vi "ADS1293_ECG.vi"() -> ()   [LabVIEW 2019]
uses:
  <vilib>/Analysis/3filter.llb/Filter Passband Type.ctl
  <vilib>/myRIO/Instrument Drivers/Onboard IO/DIO/typedefs/DIO Reference.ctl
  <vilib>/myRIO/Common/Instrument Driver Framework/Utilities/typedefs/myRIO Generic Hardware Reference.ctl
  <vilib>/myRIO/Common/Instrument Driver Framework/Utilities/typedefs/Hardware Version Enum.ctl
  <vilib>/myRIO/Common/Instrument Driver Framework/Utilities/typedefs/myRIO v1.0 Reference.ctl
  <vilib>/myRIO/Common/Instrument Driver Framework/Utilities/typedefs/Generic FPGA Reference.ctl
  <vilib>/myRIO/Common/Instrument Driver Framework/myRIO v1.0/DIO/typedefs/DIO Channels List.ctl
  <vilib>/myRIO/Common/Instrument Driver Framework/myRIO v1.0/DIO/typedefs/DIO Channels Enum.ctl
  <vilib>/userDefined/High Color/nirio_resource_hc.ctl
  <vilib>/myRIO/Instrument Drivers/Onboard IO/SPI/typedefs/SPI User Configuration.ctl
  <vilib>/myRIO/Common/Instrument Driver Framework/myRIO v1.0/SPI/typedefs/SPI Clock Phase.ctl
  <vilib>/myRIO/Common/Instrument Driver Framework/myRIO v1.0/SPI/typedefs/SPI Clock Polarity.ctl
  <vilib>/myRIO/Common/Instrument Driver Framework/myRIO v1.0/SPI/typedefs/SPI Data Direction.ctl
  <vilib>/myRIO/Common/Instrument Driver Framework/myRIO v1.0/SPI/typedefs/SPI Frame Length.ctl
  <vilib>/myRIO/Instrument Drivers/Onboard IO/SPI/typedefs/SPI Reference.ctl
  <vilib>/myRIO/Common/Instrument Driver Framework/myRIO v1.0/SPI/typedefs/SPI Channels Enum.ctl
  <vilib>/myRIO/Instrument Drivers/Onboard IO/SPI/typedefs/SPI Configuration.ctl
  <vilib>/myRIO/Common/Instrument Driver Framework/Utilities/vis/Is FPGA Ref Available.vi
  <vilib>/myRIO/Common/Instrument Driver Framework/myRIO v1.0/DIO/vis/myRIO v1.1 Open DIO.vi
  <vilib>/myRIO/Instrument Drivers/Onboard IO/DIO/vis/Write.vi
  <vilib>/myRIO/Common/Instrument Driver Framework/myRIO v1.0/SPI/vis/myRIO v1.1 Open SPI.vi
  <vilib>/myRIO/Instrument Drivers/Onboard IO/SPI/vis/Configure.vi
  <vilib>/myRIO/Instrument Drivers/Onboard IO/SPI/vis/Write.vi
  <vilib>/myRIO/Instrument Drivers/Onboard IO/SPI/vis/Read.vi
  <vilib>/myRIO/Common/Instrument Driver Framework/Utilities/vis/Validate Channels.vi
  <vilib>/myRIO/Common/Instrument Driver Framework/myRIO v1.0/DIO/vis/myRIO v1.0 Reserve DIO.vi
  <vilib>/myRIO/Common/Instrument Driver Framework/myRIO v1.0/SPI/vis/myRIO v1.0 Reserve SPI.vi
  <vilib>/myRIO/Instrument Drivers/Onboard IO/SPI/vis/Write Read.vi
  <vilib>/myRIO/Common/Instrument Driver Framework/myRIO v1.0/Resource Manager/vis/myRIO v1.0 Reserve Channel List.vi
  <vilib>/myRIO/Common/Instrument Driver Framework/myRIO v1.0/DIO/vis/myRIO v1.0 Build MUX Configuration DIO.vi
  <vilib>/myRIO/Common/Instrument Driver Framework/myRIO v1.0/SPI/vis/myRIO v1.0 Build MUX Configuration SPI.vi
  <vilib>/myRIO/Common/Instrument Driver Framework/myRIO v1.0/Resource Manager/vis/myRIO v1.0 Reserve Channel.vi
  <vilib>/myRIO/Common/Instrument Driver Framework/myRIO v1.0/Resource Manager/vis/myRIO v1.0 Unreserve Channel.vi
  <vilib>/myRIO/Common/Instrument Driver Framework/myRIO v1.0/Resource Manager/vis/myRIO v1.0 Create Configuration List.vi
  <vilib>/myRIO/Common/Instrument Driver Framework/myRIO v1.0/Resource Manager/vis/myRIO v1.0 Build Mutex Name.vi
  <vilib>/Utility/VariantDataType/GetNumericInfo.vi
  <vilib>/Utility/error.llb/Error Cluster From Error Code.vi
  <vilib>/myRIO/Common/Instrument Driver Framework/myRIO v1.0/myRIO v1.1 Open.vi
  <vilib>/myRIO/Common/Instrument Driver Framework/Utilities/vis/IO Manager.vi
  <vilib>/myRIO/Common/Instrument Driver Framework/Utilities/vis/Configuration Manager.vi
  <vilib>/myRIO/Common/Instrument Driver Framework/myRIO v1.0/Resource Manager/vis/myRIO v1.0 Configure IO.vi
  <vilib>/myRIO/Common/Instrument Driver Framework/myRIO v1.0/myRIO v1.0 Close.vi
  <vilib>/myRIO/Common/Instrument Driver Framework/myRIO v1.0/DIO/vis/myRIO v1.0 Write DIO.vi
  <vilib>/myRIO/Common/Instrument Driver Framework/myRIO v1.0/SPI/vis/myRIO v1.0 Configure SPI.vi
  <vilib>/myRIO/Common/Instrument Driver Framework/myRIO v1.0/SPI/vis/myRIO v1.0 Write Read SPI.vi
  <vilib>/myRIO/Express VI/Onboard IO/DO/DO Express VI.xnode
  <vilib>/myRIO/Instrument Drivers/Onboard IO/DIO/vis/myRIO DIO Open.xnode
  <vilib>/myRIO/Express VI/Onboard IO/SPI/SPI Express VI.xnode
  <vilib>/myRIO/Instrument Drivers/Onboard IO/SPI/vis/myRIO SPI Open.xnode
  <vilib>/Analysis/3filter.llb/FIR Windowed Filter (DBL).vi
  <vilib>/myRIO/Instrument Drivers/Onboard IO/SPI/SPI.lvlib
  <vilib>/myRIO/Instrument Drivers/Onboard IO/DIO/DIO.lvlib
  <vilib>/ptbypt/NI_PtbyPt.lvlib
  <vilib>/Analysis/NI_AALBase.lvlib
panel:
  out "OUT 2":waveform(dbl)(graph)
  in  "taps":i32=25 min=1
  in  "sampling freq: fs":dbl=1.0 format="%0.2f"
  in  "filter type":T1
  out "OUT":waveform(dbl)(graph)
  out "Waveform Channel 2":dbl[](graph)
  out "ECG DATA":u16[](array[numeric]) format="%x"
  out "Waveform Channel 1":dbl[](graph)
  out "Channel 2":u32 format="%x"
  out "Channel 1":u32 format="%x"
  in  "N":u32=6
  in  "Read Command":u16[](array[numeric])=[182, 1] format="%x"
  out "Slide":dbl(slide)=inf scale=0.0..1.0
  out "ELAPSED TIME":dbl=0.399439
  in  "SET TIME":dbl=10.0
  in  "CONFIG":u16[](array[numeric])=[0, 1] format="%x"
  in  "CH_CNFG":u16[](array[numeric])=[47, 48] format="%x"
  in  "DRDYB_SRC":u16[](array[numeric])=[39, 8] format="%x"
  in  "R3_RATE_CH2":u16[](array[numeric])=[35, 2] format="%x"
  in  "R3_RATE_CH1":u16[](array[numeric])=[34, 2] format="%x"
  in  "R2_RATE":u16[](array[numeric])=[33, 2] format="%x"
  in  "AFE_SHDN_CN":u16[](array[numeric])=[20, 36] format="%x"
  in  "OSC_CN":u16[](array[numeric])=[18, 4] format="%x"
  in  "RLD_CN":u16[](array[numeric])=[12, 4] format="%x"
  in  "CMDET_EN":u16[](array[numeric])=[10, 7] format="%x"
  in  "FLEX_CH2_CN":u16[](array[numeric])=[2, 25] format="%x"
  in  "FLEX_CH1_CN":u16[](array[numeric])=[1, 17] format="%x"
  # "INITIAL CONFIGURATIONS"
  # "3"
  # "1"
  # "2"
  # "6"
  # "4"
  # "5"
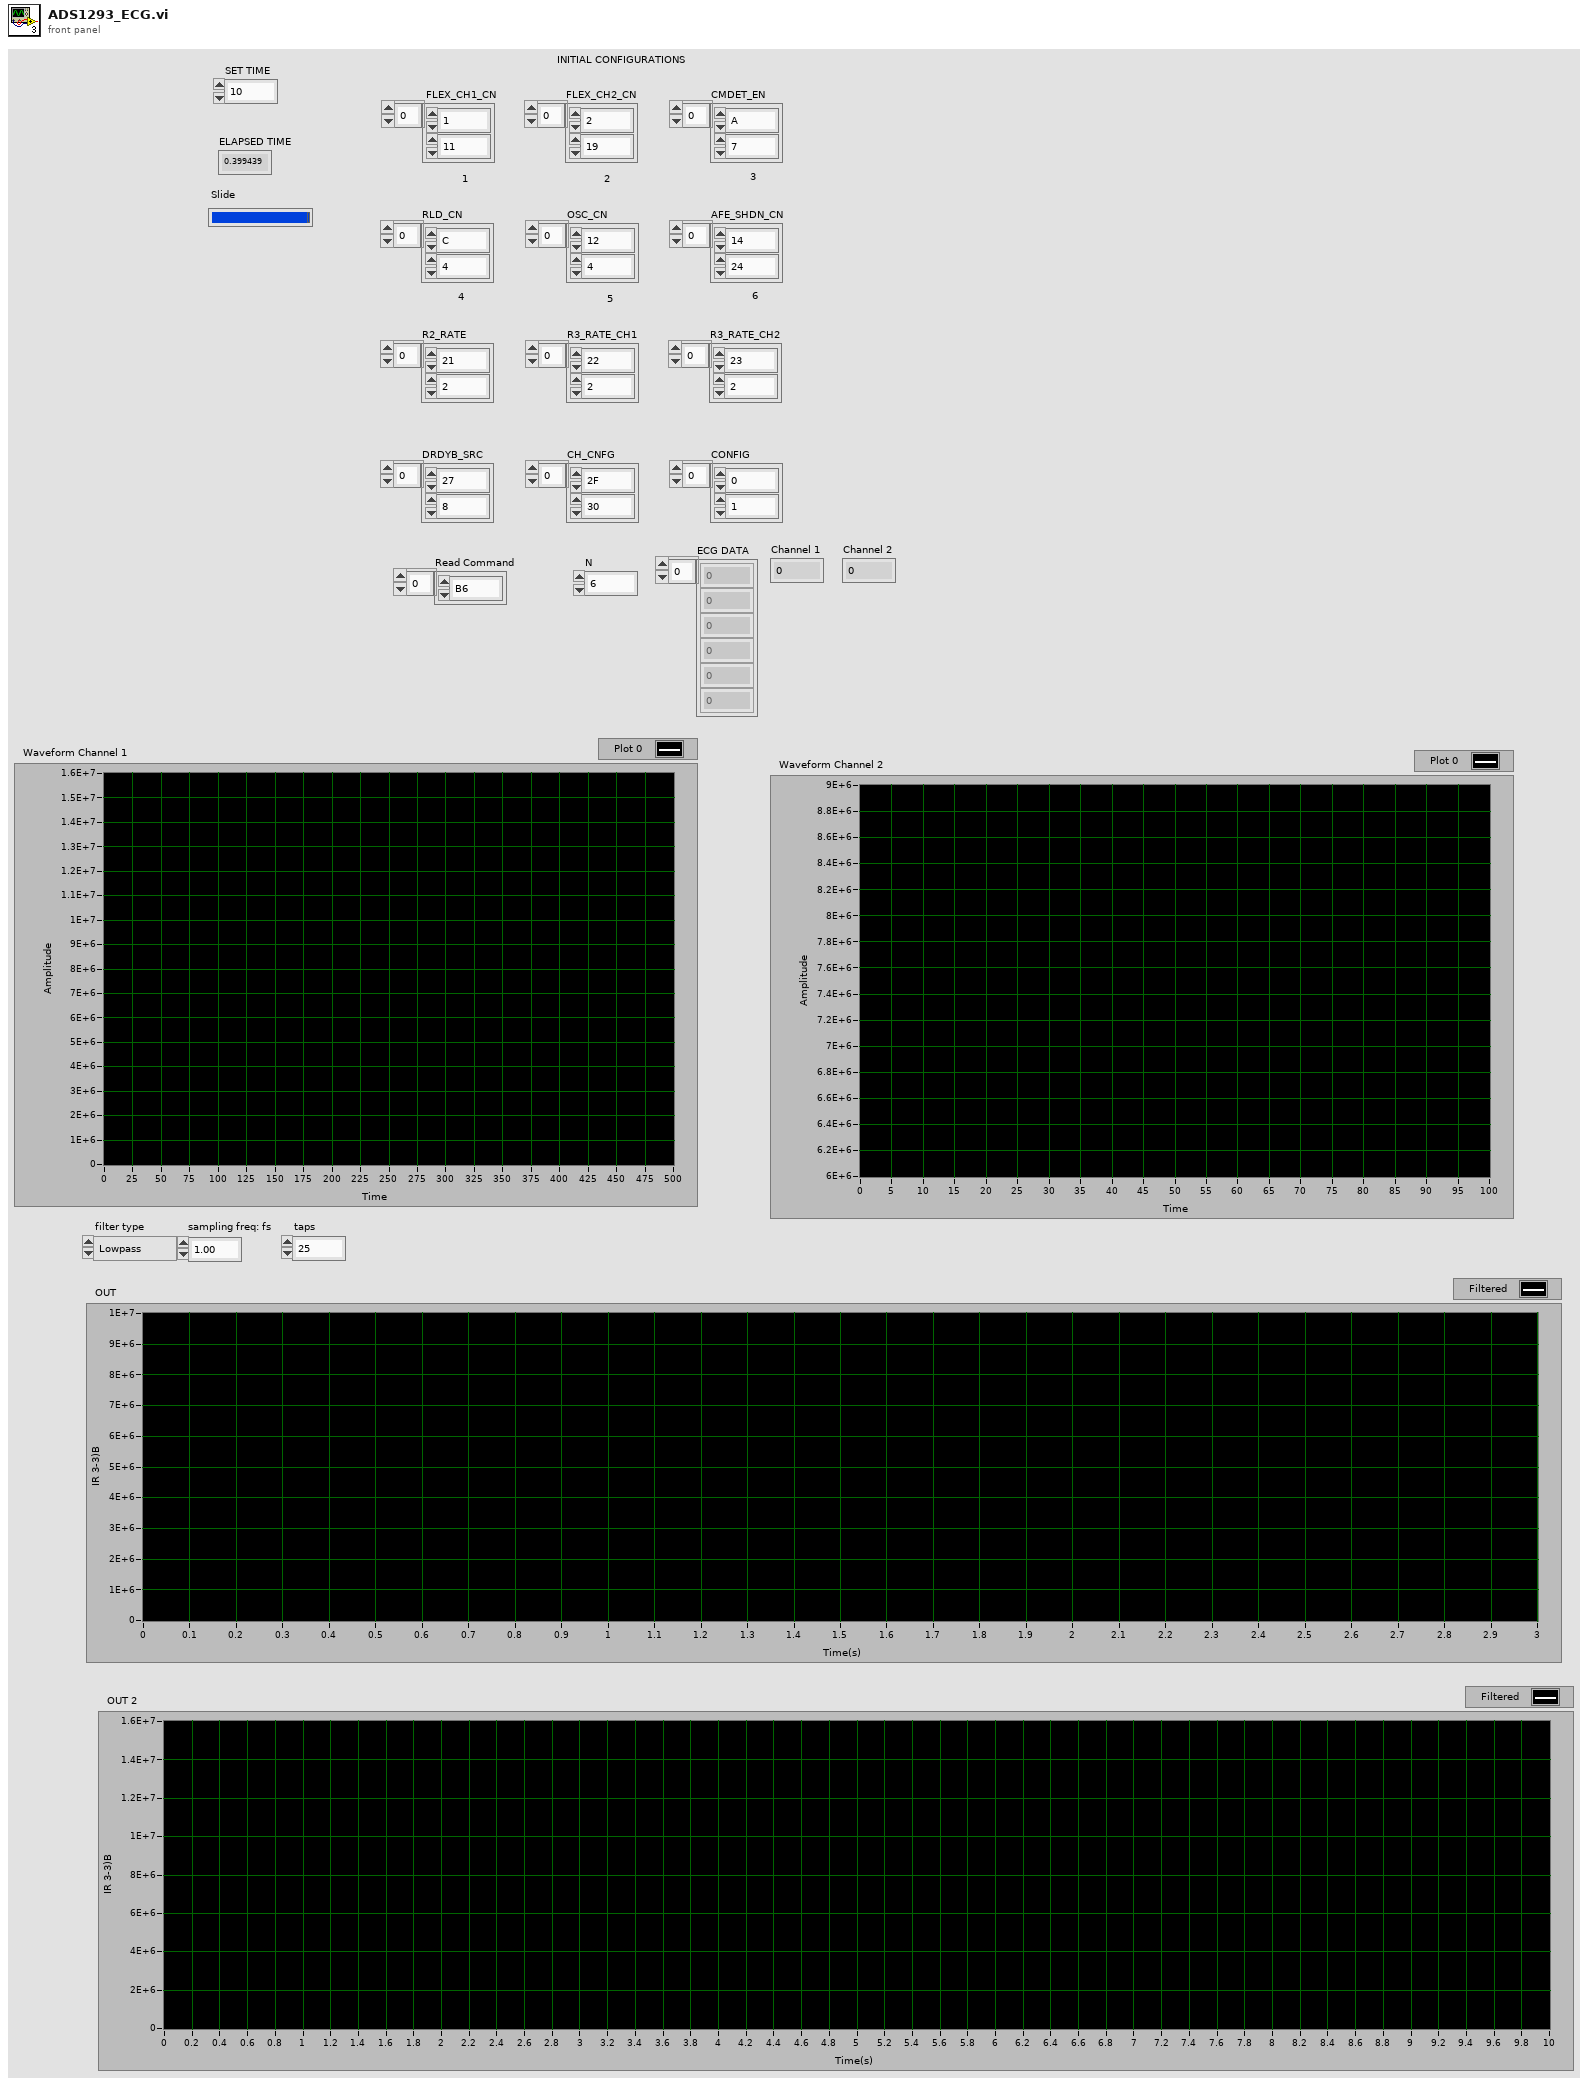
[diagram p1: front panel]
types:
  T1 = typedef "NI_AALBase.lvlib/Filter Passband Type.ctl" = enum32{"Lowpass", "Highpass", "Bandpass", "Bandstop"}
  T2 = typedef "SPI.lvlib/SPI Reference.ctl" = cluster{"myRIO Reference":T3, "SPI Channels Enum":T7, "SPI Configuration":T8}
  T3 = typedef "myRIO Generic Hardware Reference.ctl" = cluster{"myRIO Model":T4, "myRIO Hardware Reference":T5}
  T4 = typedef "Hardware Version Enum.ctl" = enum16{"Unknown", "myRIO-1900", "myRIO-1950", "roboRIO", "NI ELVIS RIO CM", "ELVIS III"}
  T5 = typedef "myRIO v1.0 Reference.ctl" = cluster{"Generic FPGA Reference":T6, "Allow multiple opens":bool}
  T6 = typedef "Generic FPGA Reference.ctl" = refnum<k20>
  T7 = typedef "SPI Channels Enum.ctl" = enum16{"Not Connected", "A/SPI", "B/SPI", "SPI/SPI"}
  T8 = typedef "SPI.lvlib/SPI Configuration.ctl" = cluster{"Frequency [Hz]":dbl, "Clock Phase":T9, "Clock Polarity":T10, "Data Direction":T11, "Frame Length":T12}
  T9 = typedef "SPI Clock Phase.ctl" = enum8{"Leading", "Trailing"}
  T10 = typedef "SPI Clock Polarity.ctl" = enum8{"Low", "High"}
  T11 = typedef "SPI Data Direction.ctl" = enum8{"Most significant bit first", "Least significant bit first"}
  T12 = typedef "SPI Frame Length.ctl" = u8
  T13 = typedef "SPI.lvlib/SPI User Configuration.ctl" = cluster{"Frequency [Hz]":dbl, "Clock Phase":T9, "Clock Polarity":T10, "Data Direction":T11, "Frame Length":T12}
  T14 = typedef "nirio_resource_hc.ctl" = tag
  T15 = typedef "DIO.lvlib/DIO Reference.ctl" = cluster{"myRIO Reference":T3, "DIO Channels List":T16}
  T16 = typedef "DIO Channels List.ctl" = T17[]
  T17 = typedef "DIO Channels Enum.ctl" = enum16{"Not Connected", "C/DIO0", "C/DIO1", "C/DIO2", "C/DIO3", "C/DIO4", "C/DIO5", "C/DIO6", "C/DIO7", "A/DIO0", "A/DIO1", "A/DIO2", "A/DIO3", "A/DIO4", "A/DIO5", "A/DIO6", "A/DIO7", "A/DIO8", "A/DIO9", "A/DIO10", "A/DIO11", "A/DIO12", "A/DIO13", "A/DIO14", "A/DIO15", "A/DIO16", "A/DIO17", "A/DIO18", "A/DIO19", "B/DIO0", "B/DIO1", "B/DIO2", "B/DIO3", "B/DIO4", "B/DIO5", "B/DIO6", "B/DIO7", "B/DIO8", "B/DIO9", "B/DIO10", "B/DIO11", "B/DIO12", "B/DIO13", "B/DIO14", "B/DIO15", "B/DIO16", "B/DIO17", "B/DIO18", "B/DIO19", "LED0", "LED1", "LED2", "LED3", "Button0", "DIO/DIO0", "DIO/DIO1", "DIO/DIO2", "DIO/DIO3", "DIO/DIO4", "DIO/DIO5", "DIO/DIO6", "DIO/DIO7", "DIO/DIO8", "DIO/DIO9", "SPI/CS0", "SPI/CS1", "SPI/CS2", "SPI/CS3", "LED RADIO (Green)", "LED RADIO (Red)", "LED COMM (Green)", "LED COMM (Red)", "LED MODE (Green)", "LED MODE (Red)"}
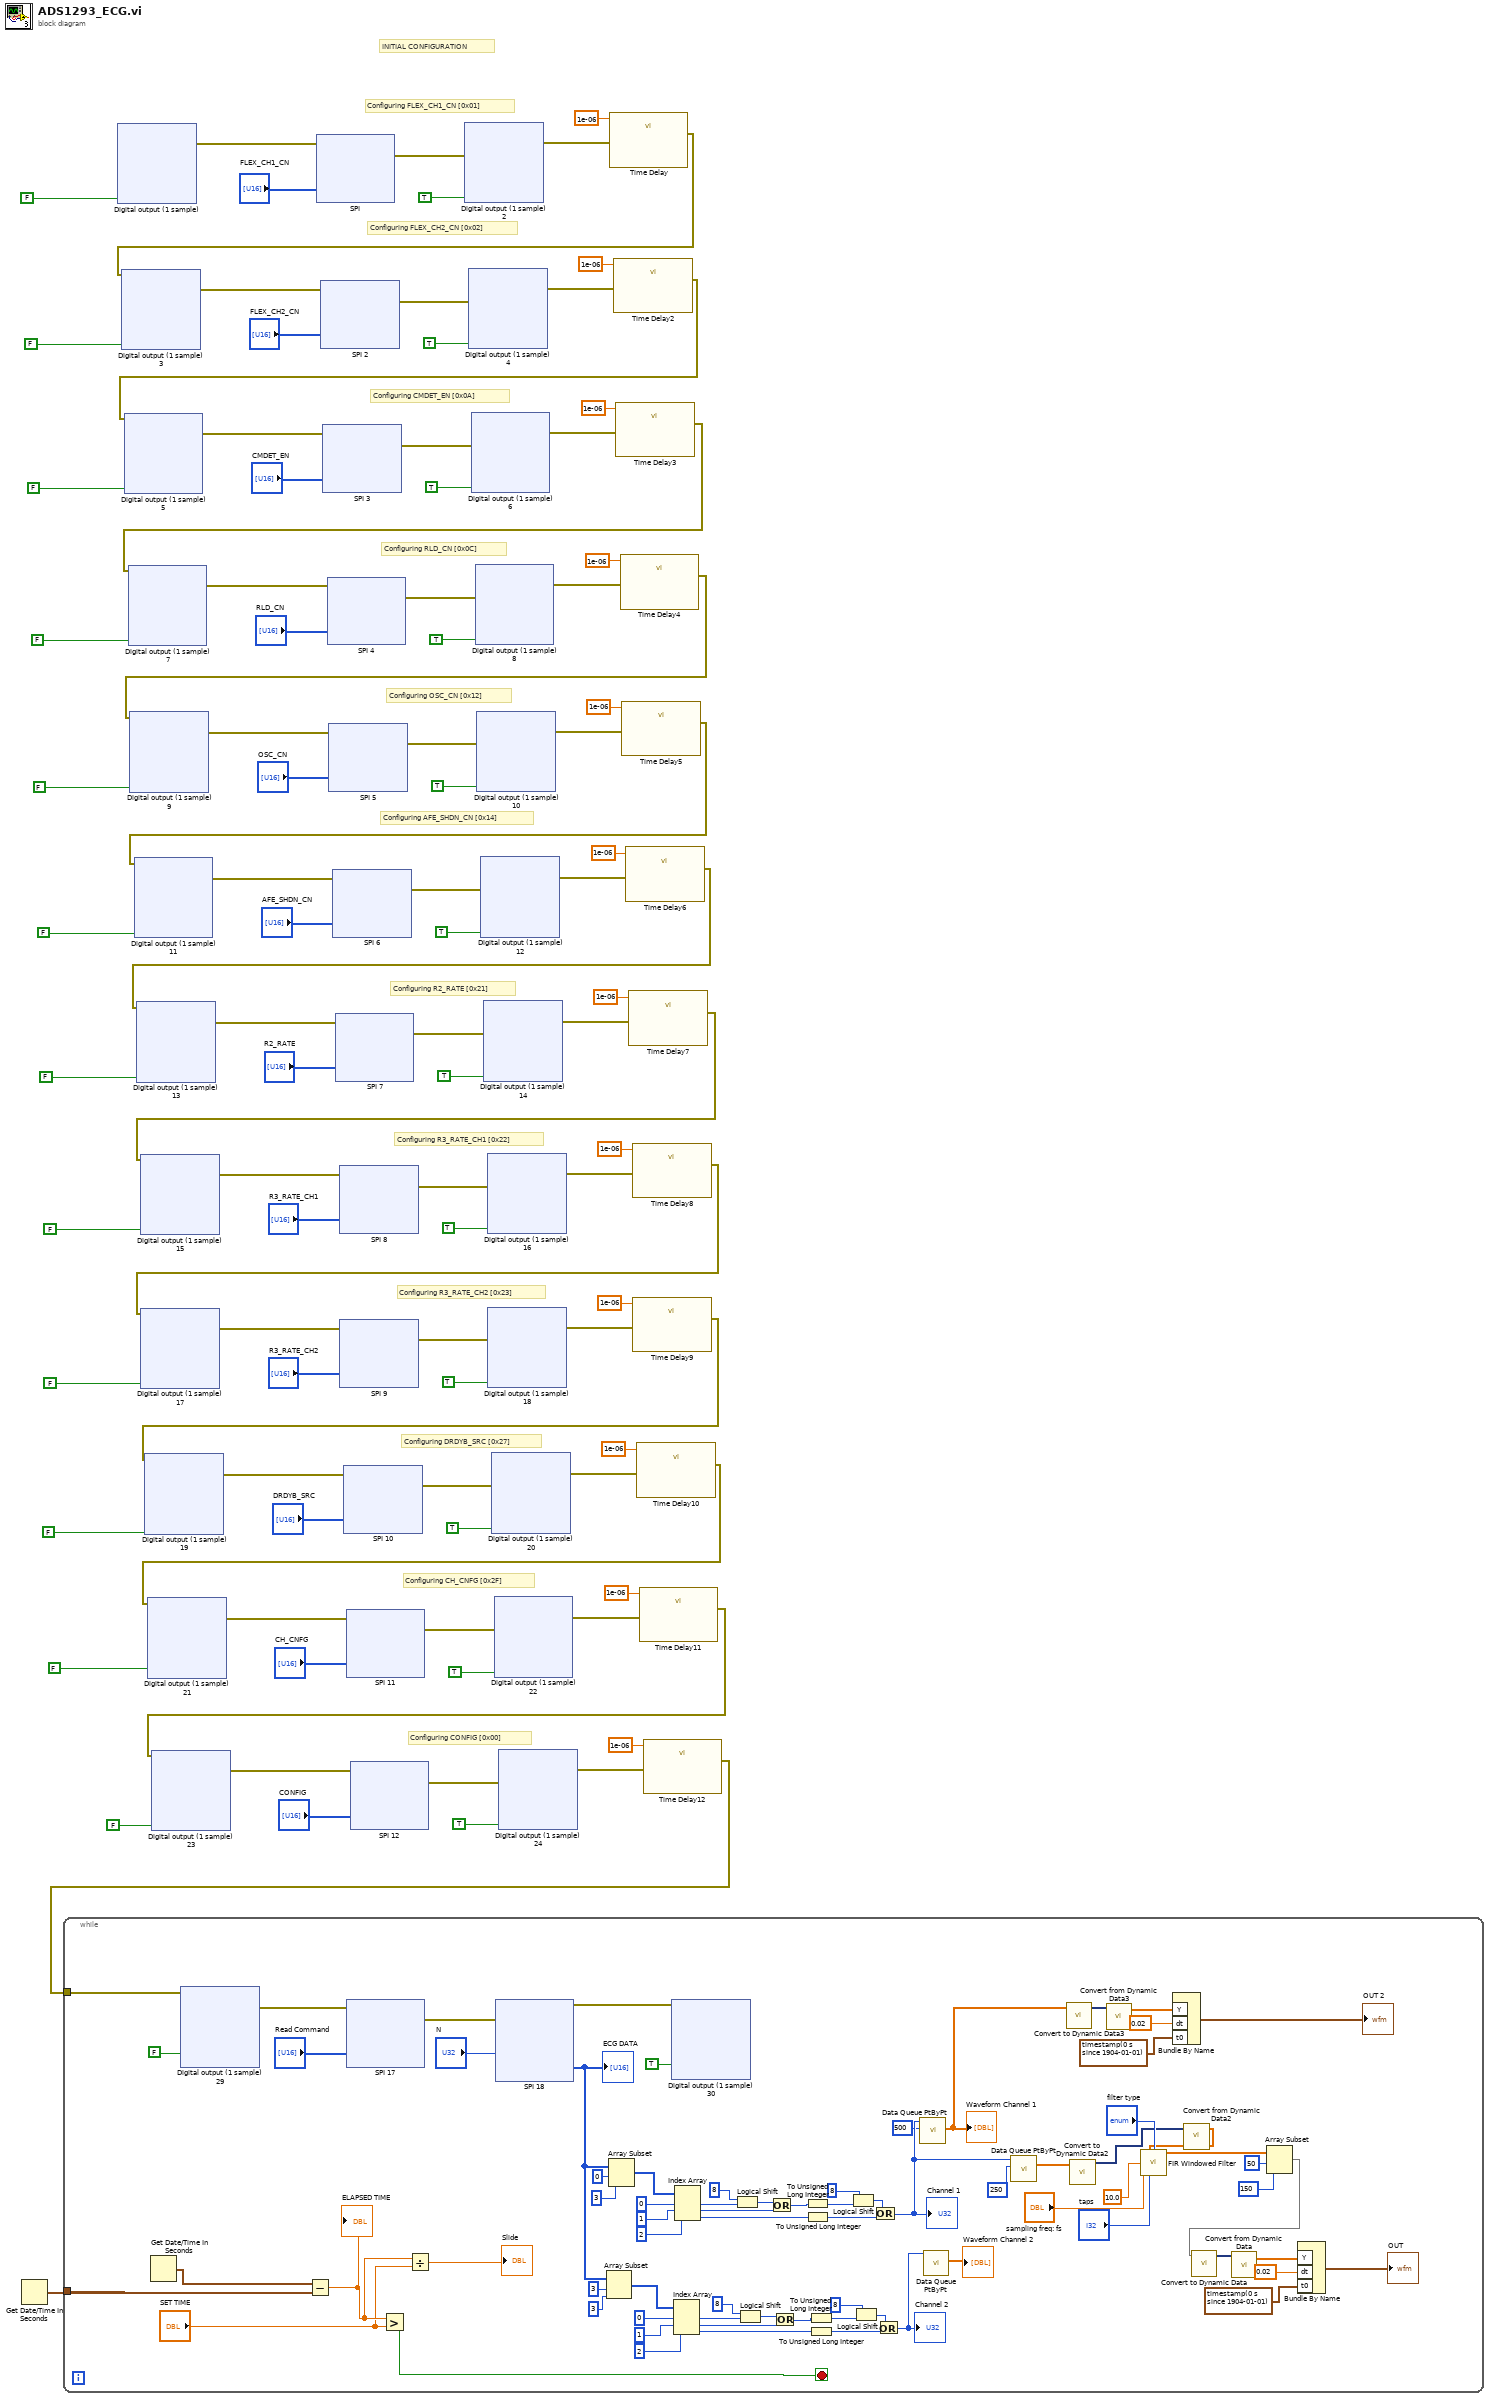
[diagram p0: block diagram]
diagram:
  # "INITIAL CONFIGURATION"
  # "Configuring CONFIG [0x00]"
  # "Configuring CH_CNFG [0x2F]"
  # "Configuring DRDYB_SRC [0x27]"
  # "Configuring R3_RATE_CH2 [0x23]"
  # "Configuring R3_RATE_CH1 [0x22]"
  # "Configuring R2_RATE [0x21]"
  # "Configuring AFE_SHDN_CN [0x14]"
  # "Configuring OSC_CN [0x12]"
  # "Configuring RLD_CN [0x0C]"
  # "Configuring CMDET_EN [0x0A]"
  # "Configuring FLEX_CH2_CN [0x02]"
  # "Configuring FLEX_CH1_CN [0x01]"
  n1 = Get Date/Time In Seconds() -> (seconds since 1Jan1904=w2:timestamp)
  n2 = xnode "Digital output (1 sample)"("A/DIO4 (Pin 19)"=FALSE) -> ("error out"=w97:errorcluster)  [unwired: 1 in]
  n3 = xnode "SPI"("Frames to Write"="FLEX_CH1_CN", "error in (no error)"=w97) -> ("error out"=w94:errorcluster)
  n4 = xnode "Digital output (1 sample) 2"("A/DIO4 (Pin 19)"=TRUE, "error in (no error)"=w94) -> ("error out"=w92:errorcluster)
  n5 = call "Time Delay"("error in (no error)"=w92, "Delay Time (s)"=1e-06) -> ("error out"=w69:errorcluster)  [unwired: 9 in]
  n6 = xnode "Digital output (1 sample) 3"("A/DIO4 (Pin 19)"=FALSE, "error in (no error)"=w69) -> ("error out"=w90:errorcluster)
  n7 = xnode "SPI 2"("Frames to Write"="FLEX_CH2_CN", "error in (no error)"=w90) -> ("error out"=w87:errorcluster)
  n8 = xnode "Digital output (1 sample) 4"("A/DIO4 (Pin 19)"=TRUE, "error in (no error)"=w87) -> ("error out"=w85:errorcluster)
  n9 = call "Time Delay2"("error in (no error)"=w85, "Delay Time (s)"=1e-06) -> ("error out"=w68:errorcluster)  [unwired: 9 in]
  n10 = xnode "Digital output (1 sample) 5"("A/DIO4 (Pin 19)"=FALSE, "error in (no error)"=w68) -> ("error out"=w83:errorcluster)
  n11 = xnode "SPI 3"("Frames to Write"="CMDET_EN", "error in (no error)"=w83) -> ("error out"=w80:errorcluster)
  n12 = xnode "Digital output (1 sample) 6"("A/DIO4 (Pin 19)"=TRUE, "error in (no error)"=w80) -> ("error out"=w78:errorcluster)
  n13 = call "Time Delay3"("error in (no error)"=w78, "Delay Time (s)"=1e-06) -> ("error out"=w67:errorcluster)  [unwired: 9 in]
  n14 = xnode "Digital output (1 sample) 7"("A/DIO4 (Pin 19)"=FALSE, "error in (no error)"=w67) -> ("error out"=w76:errorcluster)
  n15 = xnode "SPI 4"("Frames to Write"="RLD_CN", "error in (no error)"=w76) -> ("error out"=w73:errorcluster)
  n16 = xnode "Digital output (1 sample) 8"("A/DIO4 (Pin 19)"=TRUE, "error in (no error)"=w73) -> ("error out"=w71:errorcluster)
  n17 = call "Time Delay4"("error in (no error)"=w71, "Delay Time (s)"=1e-06) -> ("error out"=w3:errorcluster)  [unwired: 9 in]
  n18 = xnode "Digital output (1 sample) 9"("A/DIO4 (Pin 19)"=FALSE, "error in (no error)"=w3) -> ("error out"=w66:errorcluster)
  n19 = xnode "SPI 5"("Frames to Write"="OSC_CN", "error in (no error)"=w66) -> ("error out"=w63:errorcluster)
  n20 = xnode "Digital output (1 sample) 10"("A/DIO4 (Pin 19)"=TRUE, "error in (no error)"=w63) -> ("error out"=w61:errorcluster)
  n21 = call "Time Delay5"("error in (no error)"=w61, "Delay Time (s)"=1e-06) -> ("error out"=w38:errorcluster)  [unwired: 9 in]
  n22 = xnode "Digital output (1 sample) 11"("A/DIO4 (Pin 19)"=FALSE, "error in (no error)"=w38) -> ("error out"=w59:errorcluster)
  n23 = xnode "SPI 6"("Frames to Write"="AFE_SHDN_CN", "error in (no error)"=w59) -> ("error out"=w56:errorcluster)
  n24 = xnode "Digital output (1 sample) 12"("A/DIO4 (Pin 19)"=TRUE, "error in (no error)"=w56) -> ("error out"=w54:errorcluster)
  n25 = call "Time Delay6"("error in (no error)"=w54, "Delay Time (s)"=1e-06) -> ("error out"=w37:errorcluster)  [unwired: 9 in]
  n26 = xnode "Digital output (1 sample) 13"("A/DIO4 (Pin 19)"=FALSE, "error in (no error)"=w37) -> ("error out"=w52:errorcluster)
  n27 = xnode "SPI 7"("Frames to Write"="R2_RATE", "error in (no error)"=w52) -> ("error out"=w49:errorcluster)
  n28 = xnode "Digital output (1 sample) 14"("A/DIO4 (Pin 19)"=TRUE, "error in (no error)"=w49) -> ("error out"=w47:errorcluster)
  n29 = call "Time Delay7"("error in (no error)"=w47, "Delay Time (s)"=1e-06) -> ("error out"=w36:errorcluster)  [unwired: 9 in]
  n30 = xnode "Digital output (1 sample) 15"("A/DIO4 (Pin 19)"=FALSE, "error in (no error)"=w36) -> ("error out"=w45:errorcluster)
  n31 = xnode "SPI 8"("Frames to Write"="R3_RATE_CH1", "error in (no error)"=w45) -> ("error out"=w42:errorcluster)
  n32 = xnode "Digital output (1 sample) 16"("A/DIO4 (Pin 19)"=TRUE, "error in (no error)"=w42) -> ("error out"=w40:errorcluster)
  n33 = call "Time Delay8"("error in (no error)"=w40, "Delay Time (s)"=1e-06) -> ("error out"=w4:errorcluster)  [unwired: 9 in]
  n34 = xnode "Digital output (1 sample) 17"("A/DIO4 (Pin 19)"=FALSE, "error in (no error)"=w4) -> ("error out"=w35:errorcluster)
  n35 = xnode "SPI 9"("Frames to Write"="R3_RATE_CH2", "error in (no error)"=w35) -> ("error out"=w32:errorcluster)
  n36 = xnode "Digital output (1 sample) 18"("A/DIO4 (Pin 19)"=TRUE, "error in (no error)"=w32) -> ("error out"=w30:errorcluster)
  n37 = call "Time Delay9"("error in (no error)"=w30, "Delay Time (s)"=1e-06) -> ("error out"=w7:errorcluster)  [unwired: 9 in]
  n38 = xnode "Digital output (1 sample) 19"("A/DIO4 (Pin 19)"=FALSE, "error in (no error)"=w7) -> ("error out"=w28:errorcluster)
  n39 = xnode "SPI 10"("Frames to Write"="DRDYB_SRC", "error in (no error)"=w28) -> ("error out"=w25:errorcluster)
  n40 = xnode "Digital output (1 sample) 20"("A/DIO4 (Pin 19)"=TRUE, "error in (no error)"=w25) -> ("error out"=w23:errorcluster)
  n41 = call "Time Delay10"("error in (no error)"=w23, "Delay Time (s)"=1e-06) -> ("error out"=w6:errorcluster)  [unwired: 9 in]
  n42 = xnode "Digital output (1 sample) 21"("A/DIO4 (Pin 19)"=FALSE, "error in (no error)"=w6) -> ("error out"=w21:errorcluster)
  n43 = xnode "SPI 11"("Frames to Write"="CH_CNFG", "error in (no error)"=w21) -> ("error out"=w18:errorcluster)
  n44 = xnode "Digital output (1 sample) 22"("A/DIO4 (Pin 19)"=TRUE, "error in (no error)"=w18) -> ("error out"=w16:errorcluster)
  n45 = call "Time Delay11"("error in (no error)"=w16, "Delay Time (s)"=1e-06) -> ("error out"=w5:errorcluster)  [unwired: 9 in]
  n46 = xnode "Digital output (1 sample) 23"("A/DIO4 (Pin 19)"=FALSE, "error in (no error)"=w5) -> ("error out"=w14:errorcluster)
  n47 = xnode "SPI 12"("Frames to Write"="CONFIG", "error in (no error)"=w14) -> ("error out"=w11:errorcluster)
  n48 = xnode "Digital output (1 sample) 24"("A/DIO4 (Pin 19)"=TRUE, "error in (no error)"=w11) -> ("error out"=w9:errorcluster)
  n49 = call "Time Delay12"("error in (no error)"=w9, "Delay Time (s)"=1e-06) -> ("error out"=w1:errorcluster)  [unwired: 9 in]
  n50 = while {
    tunnel: w2 -> [w170]
    tunnel: w1 -> [w158]
    stop <- w169 stop-if-true
    n51 = Get Date/Time In Seconds() -> (seconds since 1Jan1904=w171:timestamp)
    n52 = xnode "Digital output (1 sample) 29"("A/DIO4 (Pin 19)"=FALSE, "error in (no error)"=w158) -> ("error out"=w161:errorcluster)
    n53 = Subtract(x=w171, y=w170) -> (x-y=w168:dbl)
    "ELAPSED TIME" <- w168
    n54 = xnode "SPI 17"("Frames to Write"="Read Command", "error in (no error)"=w161) -> ("error out"=w160:errorcluster)
    n55 = Greater?(x=w168, y="SET TIME") -> (0:w169:bool)
    n56 = Divide(x=w168, y="SET TIME") -> (x/y=→"Slide":dbl)
    n57 = xnode "SPI 18"("Frame Count"="N", "error in (no error)"=w160) -> ("Frames Read"=w157:u16[], "error out"=w159:errorcluster)
    "ECG DATA" <- w157
    n58 = Array Subset(array=w157, index=3, length=3) -> (w123:u16[])
    n59 = Array Subset(array=w157, index=0, length=3) -> (w101:u16[])
    n60 = xnode "Digital output (1 sample) 30"("A/DIO4 (Pin 19)"=TRUE, "error in (no error)"=w159) -> ()  [unwired: 1 out]
    n61 = Index Array(array=w123, index #1=0 ("index"), index #2=1 ("index"), index #3=2 ("index")) -> (element #1=w131:u16, element #2=w130:u16, element #3=w129:u16)
    n62 = Index Array(array=w101, index #1=0 ("index"), index #2=1 ("index"), index #3=2 ("index")) -> (element #1=w144:u16, element #2=w143:u16, element #3=w139:u16)
    n63 = Logical Shift(y=i16 8, x=w144) -> (x << y=w145:u16)
    n64 = Logical Shift(y=i16 8, x=w131) -> (x << y=w136:u16)
    n65 = Or(x=w145, y=w143) -> (x .or. y?=w142:u16)
    n66 = Or(x=w136, y=w130) -> (x .or. y?=w135:u16)
    n67 = To Unsigned Long Integer(number=w142) -> (unsigned 32bit integer=w141:u32)
    n68 = To Unsigned Long Integer(number=w139) -> (unsigned 32bit integer=w138:u32)
    n69 = To Unsigned Long Integer(number=w135) -> (unsigned 32bit integer=w134:u32)
    n70 = To Unsigned Long Integer(number=w129) -> (unsigned 32bit integer=w132:u32)
    n71 = Logical Shift(y=i16 8, x=w141) -> (x << y=w128:u32)
    n72 = Logical Shift(y=i16 8, x=w134) -> (x << y=w127:u32)
    n73 = Or(x=w128, y=w138) -> (x .or. y?=w100:u32)
    "Channel 1" <- w100
    n74 = Or(x=w127, y=w132) -> (x .or. y?=w120:u32)
    "Channel 2" <- w120
    n75 = call <vilib>:"Data Queue PtByPt.vi"("sample length"=500, "input data point"=w100) -> ("Current Queue"=w99:dbl[])  [unwired: 5 in, 4 out]
    "Waveform Channel 1" <- w99
    n76 = call <vilib>:"Data Queue PtByPt.vi"("input data point"=w120) -> ("Current Queue"=→"Waveform Channel 2":dbl[])  [unwired: 6 in, 4 out]
    n77 = call <vilib>:"Data Queue PtByPt.vi"("sample length"=250, "input data point"=w100) -> ("Current Queue"=w117:dbl[])  [unwired: 5 in, 4 out]
    n78 = call "Convert to Dynamic Data3"("Array"=w99) -> ("Dynamic Data Type"=w103:dynamicdata)  [unwired: 3 in]
    n79 = call "Convert to Dynamic Data2"("Array"=w117) -> ("Dynamic Data Type"=w113:dynamicdata)  [unwired: 3 in]
    n80 = call "Convert from Dynamic Data3"("Dynamic Data Type"=w103) -> ("Array"=w102:dbl[])  [unwired: 3 in]
    n81 = Bundle By Name("Y"=w102, "dt"=0.02, "t0"=timestamp(0 s since 1904-01-01)) -> (→"OUT 2":waveform(dbl))  [unwired: 1 in]
    n82 = call "Convert from Dynamic Data2"("Dynamic Data Type"=w113) -> ("Array"=w112:dbl[])  [unwired: 3 in]
    n83 = call-poly <vilib>:"FIR Windowed Filter.vi"("sampling freq: fs"="sampling freq: fs", "X"=w112, "filter type"="filter type", "low cutoff freq: fl"=10.0, "taps"="taps") -> ("Filtered X"=w110:dbl[])  [unwired: 9 in, 1 out]
    n84 = Array Subset(array=w110, index=50, length=150) -> (w107:dbl[])
    n85 = call "Convert to Dynamic Data"("Array"=w107) -> ("Dynamic Data Type"=w122:dynamicdata)  [unwired: 3 in]
    n86 = call "Convert from Dynamic Data"("Dynamic Data Type"=w122) -> ("Array"=w121:dbl[])  [unwired: 3 in]
    n87 = Bundle By Name("Y"=w121, "dt"=0.02, "t0"=timestamp(0 s since 1904-01-01)) -> (→"OUT":waveform(dbl))  [unwired: 1 in]
  }
